vi "Front Panel Open.vi"(8 "error in (no error)":errorcluster, 11 "UI Actor in":refnum<class "UI Actor.lvclass">) -> (0 "error out":errorcluster, 3 "UI Actor out":refnum<class "UI Actor.lvclass">)   [LabVIEW 2013, in "SET Project Editor.lvlib" / "UI Actor.lvclass"]
uses:
  UI Actor.lvclass
  UI Actor.lvclass/UI Actor.ctl
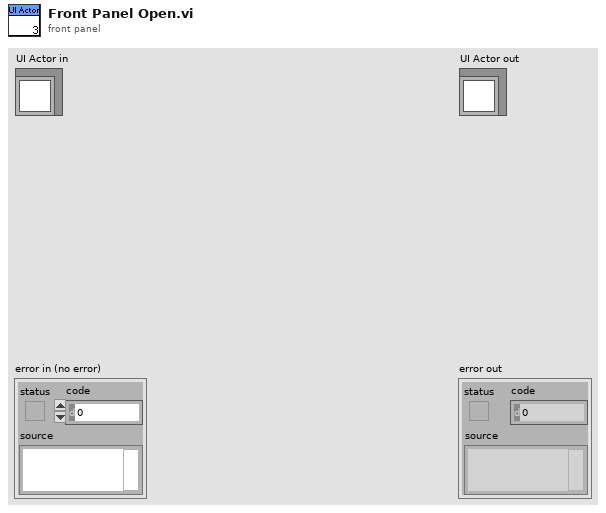
[diagram p1: front panel]
types:
  T1 = enum32{"Invalid", "Standard", "Closed", "Hidden", "Minimized", "Maximized"}
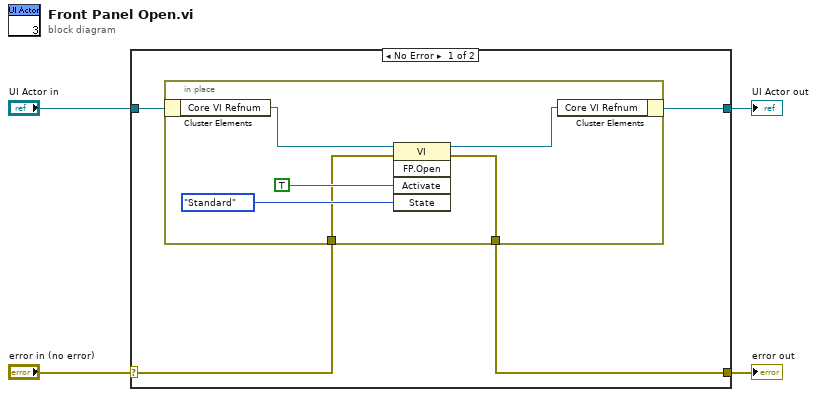
[diagram p0: block diagram]
diagram:
  n1 = case shown="No Error" "error in (no error)" {
    selector: "error in (no error)" -> [w7 w16]
    tunnel: [w8 w16] -> w3
    tunnel: [w5 w15] -> w1
    tunnel: "UI Actor in" -> [w6 w15]
    frame No Error {
      n2 = in-place {
        in-place-border: [w12] -> w8
        in-place-border: w7 -> [w11]
        n3 = in-place-cluster #1(w6) -> ("Core VI Refnum"=w10:refnum<vi>)
        n4 = invoke class="VI" method="FP.Open"(reference=w10, error in=w11, "Activate"=TRUE ("Activate?"), "State"=T1."Standard") -> (reference out=w9:refnum<vi>, error out=w12:errorcluster)  [unwired: 1 in, 3 out]
        n5 = in-place-cluster #1("Core VI Refnum"=w9) -> (w5:refnum<class "UI Actor.lvclass">)
      }
    }
    frame Error {
    }
  }
  "error out" <- w3
  "UI Actor out" <- w1
